vi "Read All Data_modified.vi"(8 "Error In":errorcluster, 11 "Leap Handle":T14) -> (0 "Error Out":errorcluster, 1 "Leap Connected?":bool, 2 "Frame":T1, 3 "Leap Handle":T14)   [LabVIEW 2015]
doc: "<b>Leap Read</b> requests and parses a <b>Frame</b> of data from the Leap Motion Controller. All the data associated with the Frame is organized into a LabVIEW cluster for accessibility.\n\nSpecifics about the data in the Frame cluster can be found by going to <b>Help » Leap Motion Controller Help</b> inside of LabVIEW"
uses:
  <vilib>/MakerHub/Leap/Private/Type Defs/Leap Handle.ctl
  C:/Program Files (x86)/National Instruments/LabVIEW 2015/vi.lib/MakerHub/Leap/Private/Libs/LeapCSharp.NET3.5.dll
  Program Files (x86)/National Instruments/LabVIEW 2015/vi.lib/MakerHub/Leap/Private/Libs/LeapCSharp.NET3.5.dll
  <vilib>/MakerHub/Leap/Private/Type Defs/Frame.ctl
  <vilib>/MakerHub/Leap/Private/Type Defs/Gesture Key Tap.ctl
  <vilib>/MakerHub/Leap/Private/Type Defs/Gesture Common.ctl
  <vilib>/MakerHub/Leap/Private/Type Defs/Gesture Type.ctl
  <vilib>/MakerHub/Leap/Private/Type Defs/Gesture State.ctl
  <vilib>/MakerHub/Leap/Private/Type Defs/Vector.ctl
  <vilib>/MakerHub/Leap/Private/Type Defs/Gesture Circle.ctl
  <vilib>/MakerHub/Leap/Private/Type Defs/Gesture Screen Tap.ctl
  <vilib>/MakerHub/Leap/Private/Type Defs/Gesture Swipe.ctl
  <vilib>/MakerHub/Leap/Private/Type Defs/Hand.ctl
  <vilib>/MakerHub/Leap/Private/Type Defs/Pointable.ctl
  <vilib>/MakerHub/Leap/Private/Type Defs/Pointable Type.ctl
  <vilib>/MakerHub/Leap/Private/Type Defs/Pointable Zone.ctl
  <vilib>/MakerHub/Leap/LMH-Leap.lvlib
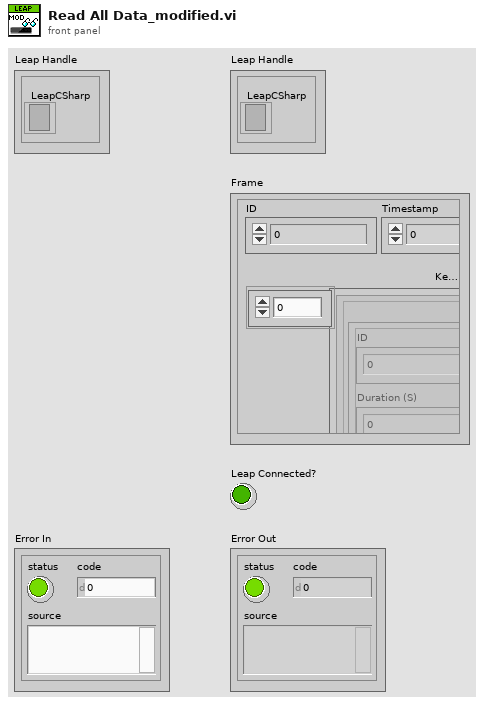
[diagram p1: front panel]
types:
  T1 = typedef "LMH-Leap.lvlib/Frame.ctl" = cluster{"ID":i64, "Timestamp":i64, "Current FPS":dbl, "Key Tap Gestures":T2[], "Circle Gestures":T7[], "Screen Tap Gestures":T8[], "Swipe Gestures":T9[], "Hands":T10[]}
  T2 = typedef "LMH-Leap.lvlib/Gesture Key Tap.ctl" = cluster{"Common":T3, "Direction":T6, "Position":T6, "Progress":dbl}
  T3 = typedef "LMH-Leap.lvlib/Gesture Common.ctl" = cluster{"ID":dbl, "Duration (S)":dbl, "Gesture Type":T4, "Gesture State":T5}
  T4 = typedef "LMH-Leap.lvlib/Gesture Type.ctl" = enum16{"Invalid", "Swipe", "Circle", "Screen Tap", "Key Tap"}
  T5 = typedef "LMH-Leap.lvlib/Gesture State.ctl" = enum16{"Invalid", "Start", "Update", "Stop"}
  T6 = typedef "LMH-Leap.lvlib/Vector.ctl" = cluster{"Pitch":sgl, "Yaw":sgl, "Roll":sgl, "Magnitude":sgl, "XYZ":sgl[]}
  T7 = typedef "LMH-Leap.lvlib/Gesture Circle.ctl" = cluster{"Common":T3, "Center":T6, "Normal":T6, "Progress":dbl, "Radius":dbl}
  T8 = typedef "LMH-Leap.lvlib/Gesture Screen Tap.ctl" = cluster{"Common":T3, "Direction":T6, "Position":T6, "Progress":dbl}
  T9 = typedef "LMH-Leap.lvlib/Gesture Swipe.ctl" = cluster{"Common":T3, "Direction":T6, "Position":T6, "Start Position":T6, "Speed":dbl}
  T10 = typedef "LMH-Leap.lvlib/Hand.ctl" = cluster{"Palm Normal":T6, "Palm Position":T6, "Palm Velocity":T6, "Direction":T6, "Palm Position (Stabilized)":T6, "Sphere Center":T6, "Pointables":T11[], "ID":i32, "Time Visible":sgl, "Sphere Radius":sgl}
  T11 = typedef "LMH-Leap.lvlib/Pointable.ctl" = cluster{"Type":T12, "Touch Zone":T13, "ID":i32, "Length":dbl, "Width":dbl, "Time Visible":dbl, "Touch Distance":dbl, "Direction":T6, "Tip Position":T6, "Tip Velocity":T6, "Tip Position (Stabilized)":T6}
  T12 = typedef "LMH-Leap.lvlib/Pointable Type.ctl" = enum16{"Finger", "Tool"}
  T13 = typedef "LMH-Leap.lvlib/Pointable Zone.ctl" = enum16{"None", "Hovering", "Touching"}
  T14 = typedef "LMH-Leap.lvlib/Leap Handle.ctl" = cluster{"LeapCSharp":refnum<k24>}
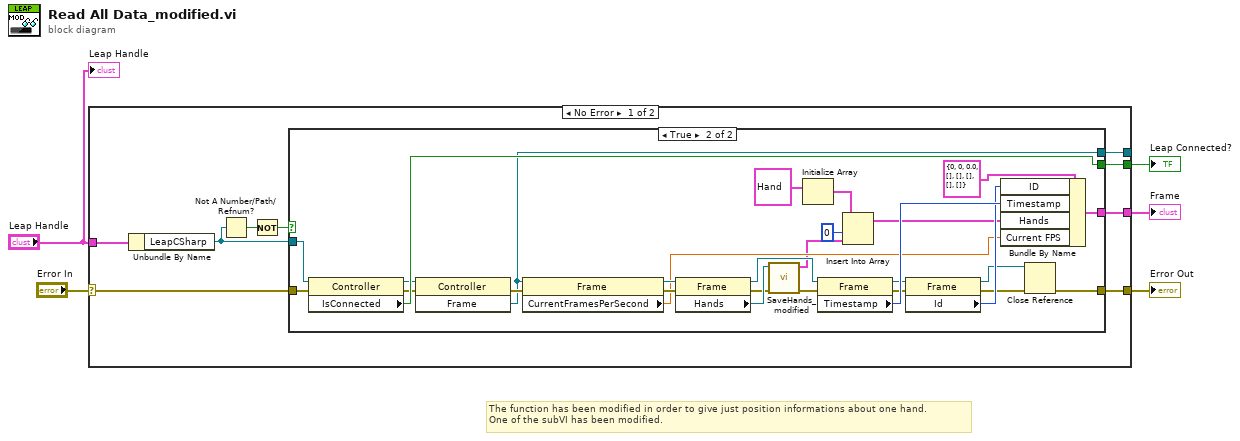
[diagram p0: block diagram]
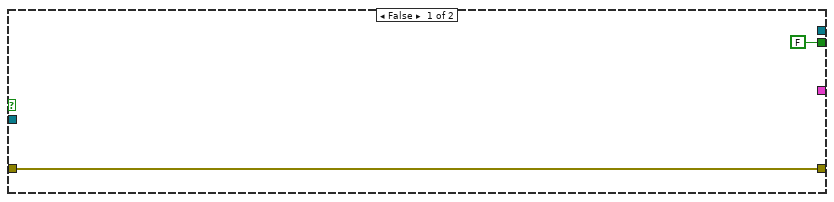
[diagram p2: hidden frame]
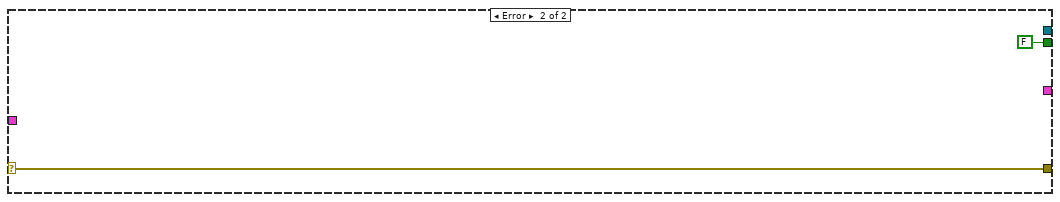
[diagram p3: hidden frame]
diagram:
  # "The function has been modified in order to give just position informations about one hand.\nOne of the subVI has been modified."
  n1 = case shown="No Error" "Error In" {
    selector: "Error In" -> [w12 w46]
    tunnel: "Leap Handle" -> [w14 _]
    tunnel: [w13 _] -> w4
    tunnel: [w11 w46] -> w2
    tunnel: [w7 FALSE ("IsConnected")] -> w1
    tunnel: [w6 _] -> _
    frame No Error {
      n2 = Unbundle By Name(w14) -> ("LeapCSharp"=w8:refnum<k24>)
      n3 = Not A Number/Path/Refnum?(number/path/refnum=w8) -> (NaN/Path/Refnum?=w10:bool)
      n4 = Not(x=w10) -> (.not. x?=w9:bool)
      n5 = case shown="True" w9 {
        tunnel: [_ w44] -> w13
        tunnel: w8 -> [_ w38]
        tunnel: w12 -> [w16 w35]
        tunnel: [w16 w42] -> w11
        tunnel: [FALSE ("IsConnected") w39] -> w7
        tunnel: [_ w28] -> w6
        frame False {
        }
        frame True {
          n6 = property class="Controller"(reference=w38, error in=w35) -> (reference out=w37:refnum<k24>, error out=w36:errorcluster, "IsConnected"=w39:bool)
          n7 = invoke class="Controller" method="Frame"(reference=w37, error in=w36) -> (error out=w34:errorcluster, "Frame"=w28:refnum<k24>)  [unwired: 1 in, 1 out]
          n8 = property class="Frame"(reference=w28, error in=w34) -> (reference out=w27:refnum<k24>, error out=w26:errorcluster, "CurrentFramesPerSecond"=w22:sgl)
          n9 = property class="Frame"(reference=w27, error in=w26) -> (reference out=w33:refnum<k24>, error out=w24:errorcluster, "Hands"=w25:refnum<k24>)
          n10 = call "SaveHands_modified.vi"("Error In"=w24, ".NET Refnum in"=w25) -> ("Error Out"=w23:errorcluster, "Left Hand"=w21:T10)  [unwired: 8 in]
          n11 = Initialize Array(T10 {"Palm Normal"={"Pitch"=0.0, "Yaw"=0.0, "Roll"=0.0, "Magnitude"=0.0, "XYZ"=[]}, "Palm Position"={"Pitch"=0.0, "Yaw"=0.0, "Roll"=0.0, "Magnitude"=0.0, "XYZ"=[]}, "Palm Velocity"={"Pitch"=0.0, "Yaw"=0.0, "Roll"=0.0, "Magnitude"=0.0, "XYZ"=[]}, "Direction"={"Pitch"=0.0, "Yaw"=0.0, "Roll"=0.0, "Magnitude"=0.0, "XYZ"=[]}, "Palm Position (Stabilized)"={"Pitch"=0.0, "Yaw"=0.0, "Roll"=0.0, "Magnitude"=0.0, "XYZ"=[]}, "Sphere Center"={"Pitch"=0.0, "Yaw"=0.0, "Roll"=0.0, "Magnitude"=0.0, "XYZ"=[]}, "Pointables"=[], "ID"=0, "Time Visible"=0.0, "Sphere Radius"=0.0} ("Hand")) -> (w17:T10[])  [unwired: 1 in]
          n12 = property class="Frame"(reference=w33, error in=w23) -> (reference out=w32:refnum<k24>, error out=w31:errorcluster, "Timestamp"=w41:i64)
          n13 = Insert Into Array(array=w17, index=0, new element=w21) -> (w20:T10[])
          n14 = property class="Frame"(reference=w32, error in=w31) -> (reference out=w29:refnum<k24>, error out=w30:errorcluster, "Id"=w40:i64)
          n15 = Bundle By Name(cluster=T1 {"ID"=0, "Timestamp"=0, "Current FPS"=0.0, "Key Tap Gestures"=[], "Circle Gestures"=[], "Screen Tap Gestures"=[], "Swipe Gestures"=[], "Hands"=[]} ("Frame"), "ID"=w40, "Timestamp"=w41, "Hands"=w20, "Current FPS"=w22) -> (w44:T1)
          n16 = Close Reference(reference=w29, error in (no error)=w30) -> (error out=w42:errorcluster)
        }
      }
    }
    frame Error {
    }
  }
  "Frame" <- w4
  "Error Out" <- w2
  "Leap Connected?" <- w1
  "Leap Handle" <- "Leap Handle"
